vi "SaveCSV2.vi"(0 "LogFileHeader":string, 1 "FCT_LOG":string, 2 "Boolean":bool, 3 "DataSave":string) -> ()   [LabVIEW 2018]
panel:
  out "concatenated string":string
  out "path":path
  out "spreadsheet string":string
  out "line string":string
  out "BufEXCEL1":string[][](array[string])
  out "line EXCEL1":string
  out "FileName":string
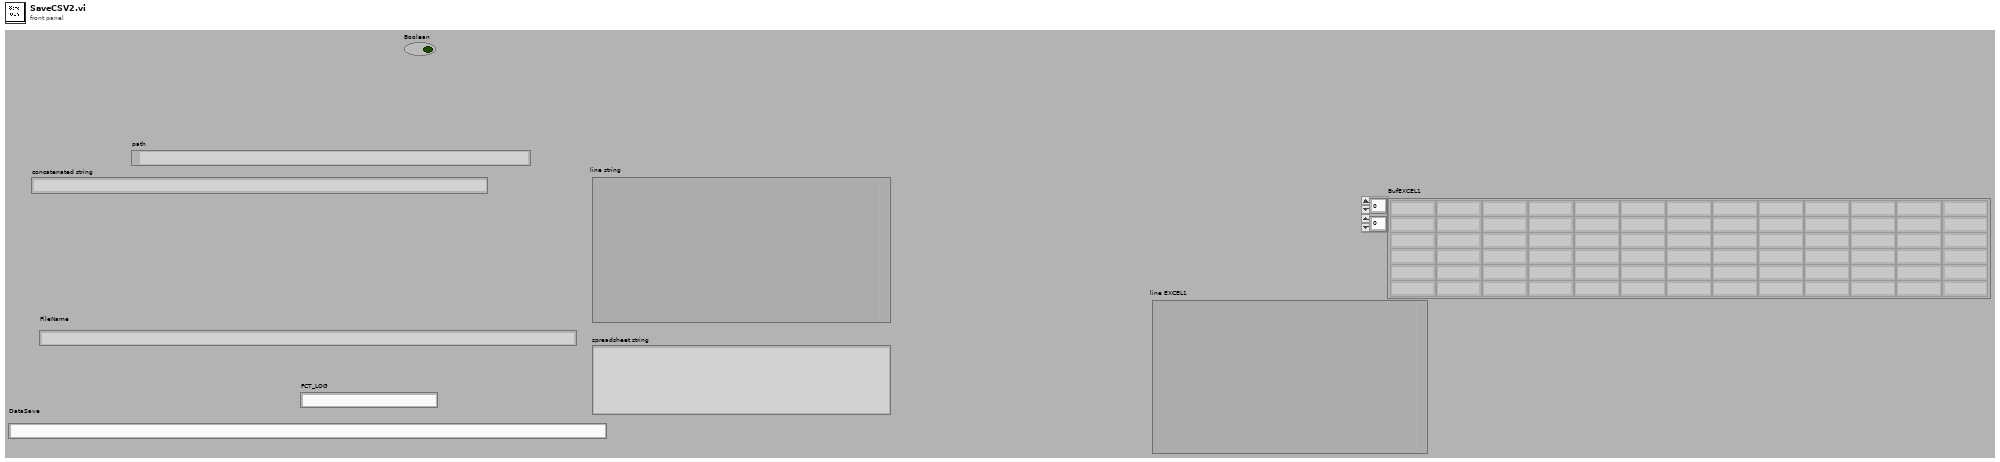
[diagram p1: front panel]
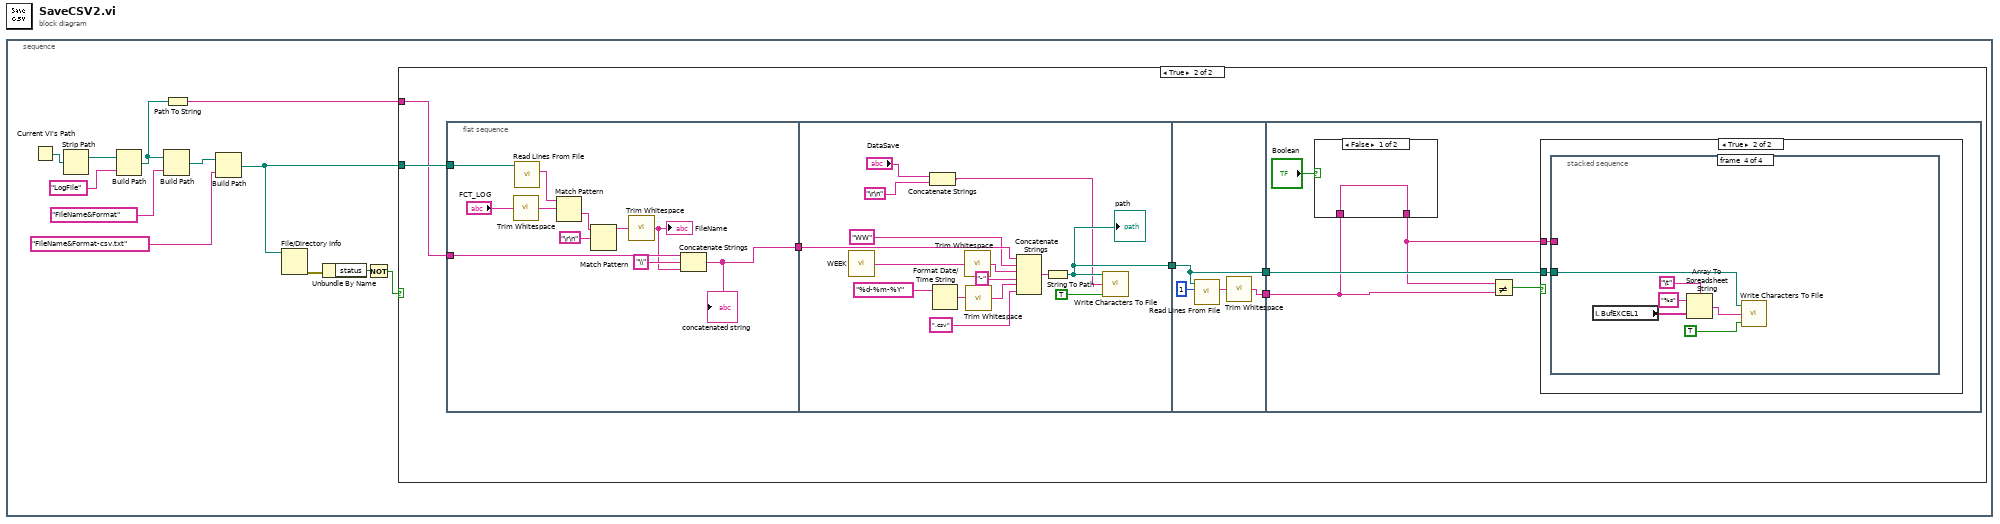
[diagram p0: block diagram]
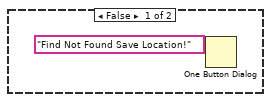
[diagram p2: hidden frame]
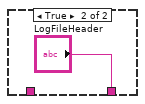
[diagram p3: hidden frame]
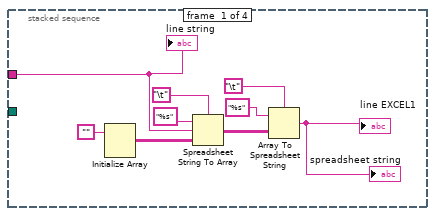
[diagram p5: hidden frame]
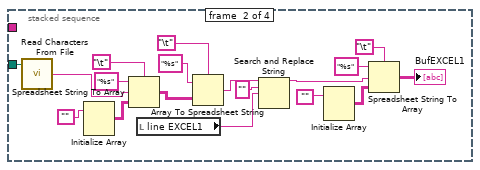
[diagram p6: hidden frame]
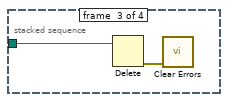
[diagram p7: hidden frame]
diagram:
  n1 = stacked-sequence {
    frame #0 {
      n2 = Current VI's Path() -> (path=w5:path)
      n3 = Strip Path(path=w5) -> (stripped path=w6:path)  [unwired: 1 out]
      n4 = Build Path(base path=w6, name or relative path="LogFile") -> (appended path=w2:path)
      n5 = Build Path(base path=w2, name or relative path="FileName&Format") -> (appended path=w9:path)
      n6 = Path To String(path=w2) -> (string=w1:string)
      n7 = Build Path(base path=w9, name or relative path="FileName&Format-csv.txt") -> (appended path=w3:path)
      n8 = File/Directory Info(path=w3) -> (error out=w12:errorcluster)  [unwired: 1 in, 6 out]
      n9 = Unbundle By Name(w12) -> ("status"=w11:bool)
      n10 = Not(x=w11) -> (.not. x?=w10:bool)
      n11 = case shown="True" w10 {
        tunnel: w3 -> [_ w19]
        tunnel: w1 -> [_ w14]
        frame False {
          n12 = One Button Dialog(message="Find Not Found Save Location!") -> ()  [unwired: 2 out]
        }
        frame True {
          n13 = flat-sequence {
            tunnel: w19 -> [w28]
            tunnel: [w22] -> w18
            tunnel: w14 -> [w23]
            tunnel: [w37] -> w17
            tunnel: w18 -> [w35]
            tunnel: w17 -> [w47]
            tunnel: [w47] -> w16
            tunnel: [w46] -> w15
            tunnel: w16 -> [w53]
            tunnel: w15 -> [w50]
            frame #0 {
              n14 = call <vilib>:"Trim Whitespace.vi"("string"="FCT_LOG") -> ("trimmed string"=w26:string)  [unwired: 1 in]
              n15 = call <vilib>:"Read Lines From File.vi"("file path (dialog if empty)"=w28) -> ("line string"=w25:string)  [unwired: 1 in, 7 out]
              n16 = Match Pattern(string=w25, regular expression=w26) -> (after substring=w30:string)  [unwired: 4 out]
              n17 = Match Pattern(string=w30, regular expression="\r\n") -> (before substring=w24:string)  [unwired: 4 out]
              n18 = call <vilib>:"Trim Whitespace.vi"("string"=w24) -> ("trimmed string"=w20:string)  [unwired: 1 in]
              "FileName" <- w20
              n19 = Concatenate Strings(w23, "\\" ("string"), w20) -> (w22:string)
              "concatenated string" <- w22
            }
            frame #1 {
              n20 = call "WEEK.vi"() -> ("WEEK"=w45:string)  [unwired: 1 out]
              n21 = Concatenate Strings("DataSave", "\r\n") -> (w33:string)
              n22 = Format Date/Time String(time format string (%c)="%d-%m-%Y") -> (date/time string=w44:string)  [unwired: 2 out]
              n23 = call <vilib>:"Trim Whitespace.vi"("string"=w45) -> ("trimmed string"=w43:string)  [unwired: 1 in]
              n24 = call <vilib>:"Trim Whitespace.vi"("string"=w44) -> ("trimmed string"=w41:string)  [unwired: 1 in]
              n25 = Concatenate Strings(w35, "WW" ("string"), w43, "-" ("string"), w41, ".csv" ("string")) -> (w38:string)
              n26 = String To Path(string=w38) -> (path=w37:path)
              "path" <- w37
              n27 = call <vilib>:"Write Characters To File.vi"("append to file? (new file:F)"=TRUE, "character string"=w33, "file path (dialog if empty)"=w37) -> ()  [unwired: 3 out]
            }
            frame #2 {
              n28 = call <vilib>:"Read Lines From File.vi"("file path (dialog if empty)"=w47, "number of lines (all:-1)"=1) -> ("line string"=w48:string)  [unwired: 7 out]
              n29 = call <vilib>:"Trim Whitespace.vi"("string"=w48) -> ("trimmed string"=w46:string)  [unwired: 1 in]
            }
            frame #3 {
              n30 = case shown="False" "Boolean" {
                tunnel: [w55 "LogFileHeader"] -> w52
                tunnel: w50 -> [w55 _]
                frame False {
                }
                frame True {
                }
              }
              n31 = Not Equal?(x=w52, y=w50) -> (x != y?=w54:bool)
              n32 = case shown="True" w54 {
                tunnel: w53 -> [_ w58]
                tunnel: w52 -> [_ w57]
                frame False {
                }
                frame True {
                  n33 = stacked-sequence {
                    tunnel: w58 -> [_ w68 w86 w90]
                    tunnel: w57 -> [w59 _ _ _]
                    frame #0 {
                      n34 = Initialize Array("") -> (w60:string[][])  [unwired: 2 out]
                      n35 = Spreadsheet String To Array(delimiter (Tab)="\t", format string="%s", spreadsheet string=w59, array type (2D Dbl)=w60) -> (array=w64:string[][])
                      n36 = Array To Spreadsheet String(delimiter (Tab)="\t", array=w64, 3:"%s" ("format string")) -> (spreadsheet string=→"line EXCEL1" →"spreadsheet string":string)
                      "line string" <- w59
                    }
                    frame #1 {
                      n37 = call <vilib>:"Read Characters From File.vi"("file path (dialog if empty)"=w68) -> ("character string"=w72:string)  [unwired: 1 in, 7 out]
                      n38 = Initialize Array("") -> (w71:string[][])  [unwired: 2 out]
                      n39 = Spreadsheet String To Array(delimiter (Tab)="\t", format string="%s", spreadsheet string=w72, array type (2D Dbl)=w71) -> (array=w74:string[][])
                      n40 = local read "line EXCEL1"() -> (w85:string)
                      n41 = Array To Spreadsheet String(delimiter (Tab)="\t", array=w74, 3:"%s" ("format string")) -> (spreadsheet string=w81:string)
                      n42 = Search and Replace String(input string=w81, search string="", replace string=w85) -> (result string=w82:string)  [unwired: 1 in, 7 out]
                      n43 = Initialize Array("") -> (w79:string[][])  [unwired: 2 out]
                      n44 = Spreadsheet String To Array(delimiter (Tab)="\t", format string="%s", spreadsheet string=w82, array type (2D Dbl)=w79) -> (array=→"BufEXCEL1":string[][])
                    }
                    frame #2 {
                      n45 = Delete(path (use dialog)=w86) -> (error out=w87:errorcluster)  [unwired: 1 in, 5 out]
                      n46 = call <vilib>:"Clear Errors.vi"("error in (no error)"=w87) -> ()  [unwired: 1 in, 6 out]
                    }
                    frame #3 {
                      n47 = local read "BufEXCEL1"() -> (w88:string[][])
                      n48 = Array To Spreadsheet String(delimiter (Tab)="\t", array=w88, 3:"%s" ("format string")) -> (spreadsheet string=w92:string)
                      n49 = call <vilib>:"Write Characters To File.vi"("append to file? (new file:F)"=TRUE, "character string"=w92, "file path (dialog if empty)"=w90) -> ()  [unwired: 3 out]
                    }
                  }
                }
              }
            }
          }
        }
      }
    }
  }
